vi "Get Row as String Array.vi"(8 "error in (no error)":errorcluster, 10 "Preserve DB Column Order (F)":bool, 11 "Table in":refnum<class "Table.lvclass">) -> (0 "error out":errorcluster, 1 "Row Values":string[](array[string]), 2 "Column Names":string[](array[string]), 3 "Table out":refnum<class "Table.lvclass">)   [LabVIEW 2020, in "Table.lvlib" / "Table.lvclass"]
uses:
  Table.lvclass
  Table.lvclass/Table.ctl
  Column Interface/Column Interface Class/Column Interface.lvclass
  Table Configuration Interface/Table Configuration Interface.lvclass
  Database Interfaces/Database Interface Class/Database Interface.lvclass
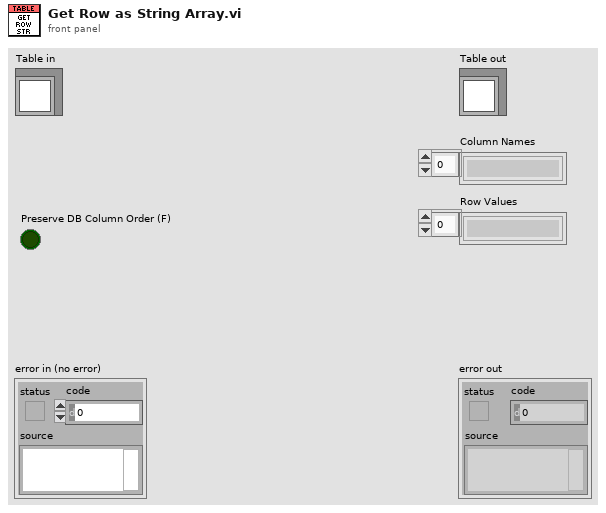
[diagram p1: front panel]
types:
  T1 = map{string, refnum<class "Column Interface.lvclass">}
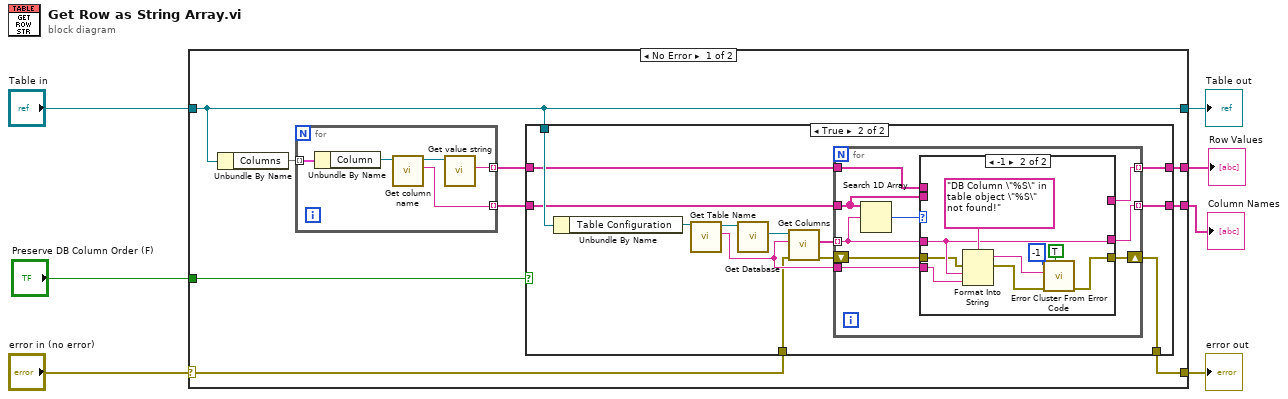
[diagram p0: block diagram]
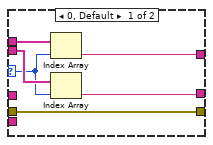
[diagram p3: hidden frame]
diagram:
  n1 = case shown="No Error" "error in (no error)" {
    selector: "error in (no error)" -> [w8 w63]
    tunnel: [w9 w63] -> w6
    tunnel: [w10 w62] -> w4
    tunnel: "Table in" -> [w10 w62]
    tunnel: [w11 _] -> w3
    tunnel: [w12 _] -> w2
    tunnel: "Preserve DB Column Order (F)" -> [w15 _]
    frame No Error {
      n2 = Unbundle By Name(w10) -> ("Columns"=w16:T1)
      n3 = for {
        tunnel: w16 -> [w60] mode=indexing
        tunnel: [w58] -> w13 mode=indexing
        tunnel: [w57] -> w14 mode=indexing
        n4 = Unbundle By Name(w60) -> ("Column"=w59:refnum<class "Column Interface.lvclass">)
        n5 = call-dynamic "Get column name.vi"("Column Interface in"=w59) -> ("Name"=w58:string, "Column Interface out"=w61:refnum<class "Column Interface.lvclass">)  [unwired: 8 in, 1 out]
        n6 = call-dynamic "Get value string.vi"("Column Interface in"=w61) -> ("Value"=w57:string)  [unwired: 8 in, 2 out]
      }
      n7 = case shown="True" w15 {
        tunnel: w14 -> [w19 w26]
        tunnel: w13 -> [w18 w27]
        tunnel: [w19 w25] -> w12
        tunnel: [w18 w24] -> w11
        tunnel: w10 -> [_ w32]
        tunnel: [w17 w21] -> w9
        tunnel: w8 -> [w17 w20]
        frame False {
        }
        frame True {
          n8 = Unbundle By Name(w32) -> ("Table Configuration"=w31:refnum<class "Table Configuration Interface.lvclass">)
          n9 = call-dynamic "Get Table Name.vi"("Table Configuration Interface in"=w31) -> ("Table Name"=w23:string, "Table Configuration Interface out"=w30:refnum<class "Table Configuration Interface.lvclass">)  [unwired: 8 in, 1 out]
          n10 = call-dynamic "Get Database.vi"("Table Configuration Interface in"=w30) -> ("Database"=w29:refnum<class "Database Interface.lvclass">)  [unwired: 8 in, 2 out]
          n11 = call-dynamic "Get Columns.vi"("error in (no error)"=w20, "Table Name"=w23, "Database Interface in"=w29) -> ("error out"=w22:errorcluster, "Column Name Array"=w28:string[])  [unwired: 6 in, 1 out]
          n12 = for {
            tunnel: w28 -> [w36] mode=indexing
            tunnel: w27 -> [w39]
            tunnel: w26 -> [w40]
            tunnel: [w38] -> w25 mode=indexing
            tunnel: [w37] -> w24 mode=indexing
            tunnel: w23 -> [w35]
            shift-right: [w33] -> w21
            shift-left: w22 -> [w34]
            n13 = Search 1D Array(1D array=w39, element=w36) -> (index of element=w41:i32)  [unwired: 1 in]
            n14 = case shown="-1" w41 {
              selector: w41 -> [w45 _]
              tunnel: w40 -> [w47 _]
              tunnel: w39 -> [w46 _]
              tunnel: [w44 _] -> w38
              tunnel: [w43 w55] -> w37
              tunnel: w36 -> [_ w55]
              tunnel: w35 -> [_ w54]
              tunnel: w34 -> [w42 w51]
              tunnel: [w42 w48] -> w33
              frame 0, Default {
                n15 = Index Array(array=w47, index=w45) -> (element=w44:string)
                n16 = Index Array(array=w46, index=w45) -> (element=w43:string)
              }
              frame -1 {
                n17 = Format Into String(format string="DB Column \"%S\" in table object \"%S\" not found!", error in=w51, w55, w54) -> (resulting string=w50:string, error out=w49:errorcluster)  [unwired: 1 in]
                n18 = call <vilib>:"Error Cluster From Error Code.vi"("show call chain? (False)"=TRUE, "error in (no error)"=w49, "error message (\"\")"=w50, "error code (0)"=-1) -> ("error out"=w48:errorcluster)  [unwired: 5 in]
              }
            }
          }
        }
      }
    }
    frame Error {
    }
  }
  "error out" <- w6
  "Table out" <- w4
  "Column Names" <- w3
  "Row Values" <- w2
